vi "get_settings_cluster.vi"(8 "error in (no error)":errorcluster, 11 "GenericPlugin in":refnum<class "DetectorYK090623DAQmxAnalog.lvclass">) -> (0 "error out":errorcluster, 2 "settings cluster":variant, 3 "GenericPlugin out":refnum<class "DetectorYK090623DAQmxAnalog.lvclass">)   [LabVIEW 2010, in "DetectorYK090623DAQmxAnalog.lvclass"]
uses:
  DetectorYK090623DAQmxAnalog.lvclass
  DetectorYK090623DAQmxAnalog.lvclass/DetectorYK090623DAQmxAnalog.ctl
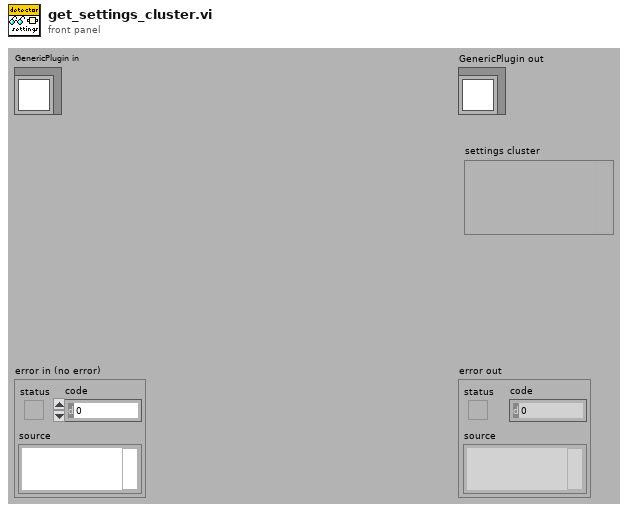
[diagram p1: front panel]
types:
  T1 = typedef "DetectorYK090623DAQmxAnalog.lvclass/settings_cluster.ctl" = cluster{"voltaqe":dbl[unit]}
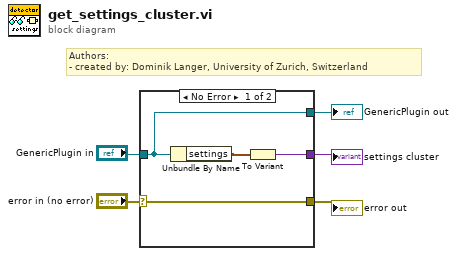
[diagram p0: block diagram]
diagram:
  # "Authors: \n- created by: Dominik Langer, University of Zurich, Switzerland"
  n1 = case shown="No Error" "error in (no error)" {
    selector: "error in (no error)" -> [w9 w10]
    tunnel: [w9 w10] -> w4
    tunnel: [w8 w11] -> w3
    tunnel: "GenericPlugin in" -> [w8 w11]
    tunnel: [w6 _] -> w1
    frame No Error {
      n2 = Unbundle By Name(w8) -> ("settings"=w7:T1)
      n3 = To Variant(anything=w7) -> (Variant=w6:variant)
    }
    frame Error {
    }
  }
  "error out" <- w4
  "GenericPlugin out" <- w3
  "settings cluster" <- w1
